vi "chargepulse.vi"(0 "Battery Detect Voltage (0V)":dbl format="%#.6g", 1 "VISA resource name":refnum<visa-resource-name>, 2 "Path":path, 3 "DAQmx Task Name":refnum<k21>, 5 "Voltage Setpoint (0 V)":dbl format="%#.6g", 9 "Current Setpoint (0 A)":dbl format="%#.6g", 11 "Power Setpoint (0 W)":dbl format="%#.6g", 12 "error in (no error)":errorcluster, 13 "Task error in":errorcluster, 14 "pulse time":dbl) -> (4 "VISA resource name out":refnum<visa-resource-name>, 6 "Filename Out":path, 8 "task out":refnum<k21>, 10 "error out":errorcluster, 15 "Task error out":errorcluster)   [LabVIEW 2020]
uses:
  <vilib>/DAQmx/read.llb/DAQmx Read (Analog 1D DBL NChan 1Samp).vi
  <vilib>/DAQmx/miscellaneous.llb/DAQmx Fill In Error Info.vi
  <instrlib>/NH Research Regenerative Test Series/Public/Data/Read (Ave Current).vi
  <instrlib>/NH Research Regenerative Test Series/Public/Data/Low Level/Fetch (Ave Voltage).vi
  <instrlib>/NH Research Regenerative Test Series/Public/Data/Low Level/Fetch (Ave True Power).vi
  <instrlib>/NH Research Regenerative Test Series/NH Research Regenerative Test Series.lvlib
panel:
  out "Ave Current (A)":dbl
  out "Ave Voltage (V)":dbl
  out "Ave True Power (W)":dbl
  out "Status Byte Register":T1
  in  "Logical Instrument Number":u32=1
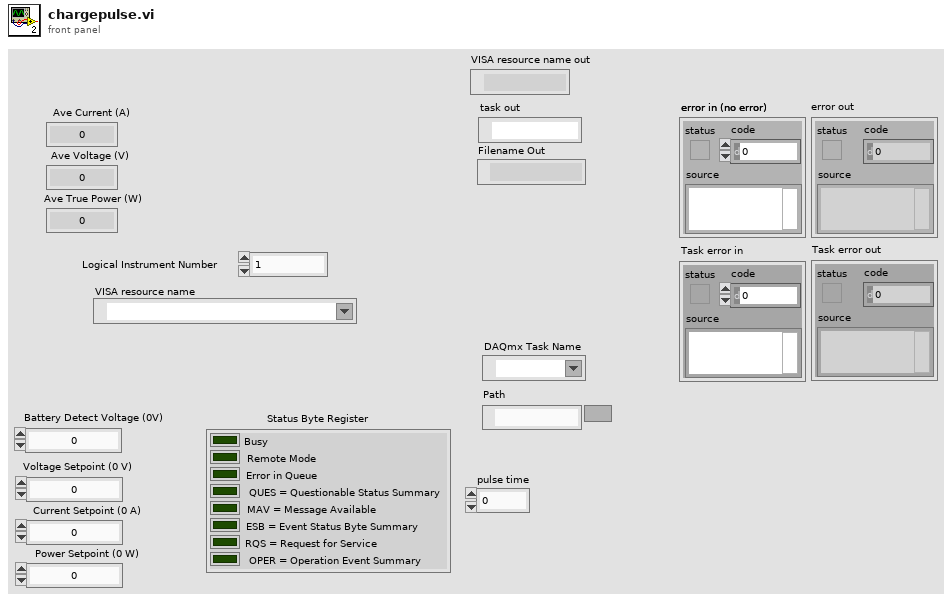
[diagram p1: front panel]
types:
  T1 = cluster{"Busy":bool, "Remote Mode":bool, "Error in Queue":bool, "QUES = Questionable Status Summary":bool, "MAV = Message Available":bool, "ESB = Event Status Byte Summary":bool, "RQS = Request for Service":bool, "OPER = Operation Event Summary":bool}
  T2 = cluster{"data[0]":dbl, "data[1]":dbl, "data[2]":dbl, "data[3]":dbl, "data[4]":dbl, "data[5]":dbl, "data[6]":dbl, "data[7]":dbl, "data[8]":dbl}
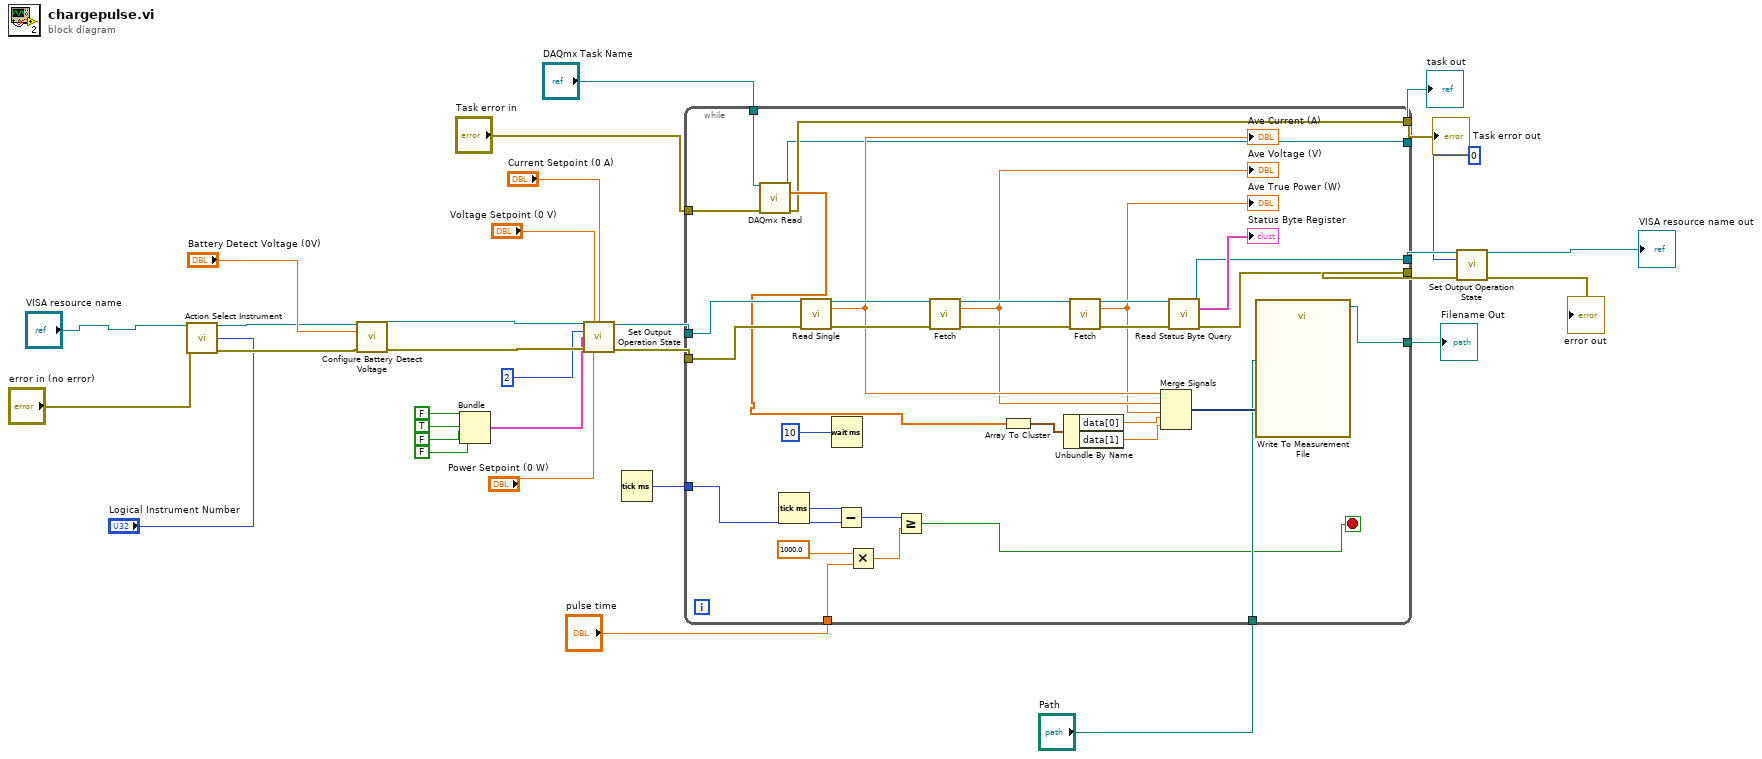
[diagram p0: block diagram]
diagram:
  n1 = call <instrlib>:"Action Select Instrument.vi"("VISA resource name"="VISA resource name", "Logical Instrument Number"="Logical Instrument Number", "error in (no error)"="error in (no error)") -> ("VISA resource name out"=w28:refnum<visa-resource-name>, "error out"=w27:errorcluster)  [unwired: 11 in]
  n2 = call <vilib>:"Configure Battery Detect Voltage.vi"("VISA resource name"=w28, "Battery Detect Voltage (0V)"="Battery Detect Voltage (0V)", "error in (no error)"=w27) -> ("VISA resource name out"=w26:refnum<visa-resource-name>, "error out"=w25:errorcluster)  [unwired: 11 in]
  n3 = Bundle(FALSE, TRUE, FALSE, FALSE) -> (w12:cluster{bool, bool, bool, bool})  [unwired: 1 in]
  n4 = call <vilib>:"Set Output Operation State.vi"("VISA resource name"=w26, "Voltage Setpoint (0 V)"="Voltage Setpoint (0 V)", "Current Setpoint (0 A)"="Current Setpoint (0 A)", "Mode (0: Off)"=2, "Enable"=w12, "error in (no error)"=w25, "Power Setpoint (0 W)"="Power Setpoint (0 W)") -> ("VISA resource name out"=w21:refnum<visa-resource-name>, "error out"=w20:errorcluster)  [unwired: 7 in]
  n5 = Tick Count (ms)() -> (millisecond timer value=w8:u32)
  n6 = while {
    tunnel: w21 -> [w58]
    tunnel: w20 -> [w57]
    tunnel: [w55] -> w24
    tunnel: [w54] -> w23
    tunnel: "pulse time" -> [w37]
    tunnel: "Path" -> [w49]
    tunnel: "DAQmx Task Name" -> [w48]
    tunnel: w8 -> [w38]
    tunnel: [w36] -> w7
    tunnel: [w35] -> w6
    tunnel: [w34] -> w5
    tunnel: "Task error in" -> [w33]
    stop <- w39 stop-if-true
    n7 = call-poly <vilib>:"DAQmx Read.vi"("task/channels in"=w48, "error in"=w33) -> ("task out"=w35:refnum<k21>, "data"=w47:dbl[], "error out"=w36:errorcluster)  [unwired: 11 in]
    n8 = Tick Count (ms)() -> (millisecond timer value=w43:u32)
    n9 = call-poly <instrlib>:"Read Single.vi"("VISA resource name"=w58, "error in (no error)"=w57) -> ("VISA resource name out"=w63:refnum<visa-resource-name>, "Ave Current (A)"=w53:dbl, "error out"=w64:errorcluster)  [unwired: 11 in]
    "Ave Current (A)" <- w53
    n10 = Wait (ms)(milliseconds to wait=10) -> ()  [unwired: 1 out]
    n11 = Subtract(x=w43, y=w38) -> (x-y=w40:u32)
    n12 = Multiply(x=1000.0, y=w37) -> (x*y=w41:dbl)
    n13 = Greater Or Equal?(x=w40, y=w41) -> (x >= y?=w39:bool)
    n14 = call-poly <instrlib>:"Fetch.vi"("VISA resource name"=w63, "error in (no error)"=w64) -> ("VISA resource name out"=w62:refnum<visa-resource-name>, "Ave Voltage (V)"=w52:dbl, "error out"=w61:errorcluster)  [unwired: 11 in]
    "Ave Voltage (V)" <- w52
    n15 = Array To Cluster(array=w47) -> (cluster=w46:T2)
    n16 = Unbundle By Name(w46) -> ("data[0]"=w45:dbl, "data[1]"=w44:dbl)
    n17 = call-poly <instrlib>:"Fetch.vi"("VISA resource name"=w62, "error in (no error)"=w61) -> ("VISA resource name out"=w60:refnum<visa-resource-name>, "Ave True Power (W)"=w51:dbl, "error out"=w59:errorcluster)  [unwired: 11 in]
    "Ave True Power (W)" <- w51
    n18 = Merge Signals "Merge Signals"(w53, w52, w51, w45, w44) -> (w65:dynamicdata)
    n19 = call <instrlib>:"Read Status Byte Query.vi"("VISA resource name"=w60, "error in (no error)"=w59) -> ("VISA resource name out"=w55:refnum<visa-resource-name>, "Status Byte Register"=→"Status Byte Register":T1, "error out"=w54:errorcluster)  [unwired: 11 in]
    n20 = call "Write To Measurement File"("Signals"=w65, "Filename"=w49) -> ("Filename Out"=w34:path)  [unwired: 15 in, 2 out]
  }
  "Task error out" <- w7
  "task out" <- w6
  "Filename Out" <- w5
  n21 = call <vilib>:"Set Output Operation State.vi"("VISA resource name"=w24, "Mode (0: Off)"=0, "error in (no error)"=w23) -> ("VISA resource name out"=→"VISA resource name out":refnum<visa-resource-name>, "error out"=→"error out":errorcluster)  [unwired: 11 in]
